vi "Take Measurement.vi"(8 "error in (no error)":errorcluster, 11 "SweepControl in":refnum<class "Sweep Control.lvclass">) -> (0 "error out":errorcluster, 3 "SweepControl":refnum<class "Sweep Control.lvclass">)   [LabVIEW 2019, in "Sweep Control.lvclass"]
uses:
  Sweep Control.lvclass
  Sweep Control.lvclass/Sweep Control.ctl
  <userlib>/LevyLab/Transport/Transport/Transport.lvclass/Transport.ctl
  <userlib>/LevyLab/Transport/Transport/Transport.lvclass
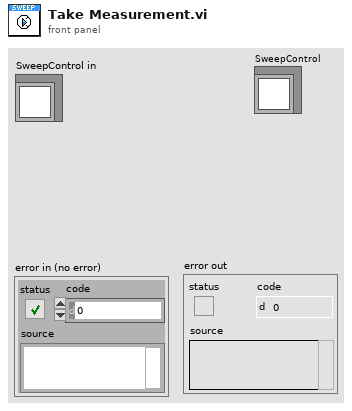
[diagram p1: front panel]
types:
  T1 = typedef "Sweep Control.lvclass/Enum - Experiments.ctl" = enum16{"Lockin_time", "Lockin_sweep", "Lockin_DelayLine"}
  T2 = typedef "Transport.lvclass/Lockin_Sweep JSON--Cluster.ctl" = cluster{"Sweep Time (s)":dbl, "Initial Wait (s)":dbl, "Return to Start":bool, "Sweep Channels":T3, "Sweep Tables":cluster{"Ch":i32, "Table":dbl[]}[]}
  T3 = typedef "Instrument.DAQ.lvclass/Sweep.Channel--Cluster--Array.ctl" = T4[]
  T4 = typedef "Instrument.DAQ.lvclass/Sweep.Channel--Cluster.ctl" = cluster{"Enable?":bool, "Channel":u16, "Start":dbl, "End":dbl, "Pattern":T5, "Table":dbl[]}
  T5 = typedef "Instrument.DAQ.lvclass/Sweep.Pattern--Enum.ctl" = enum16{"Ramp /", "Ramp /\\", "Smooth Ramp _/", "Smooth Ramp _/\\_", "Table"}
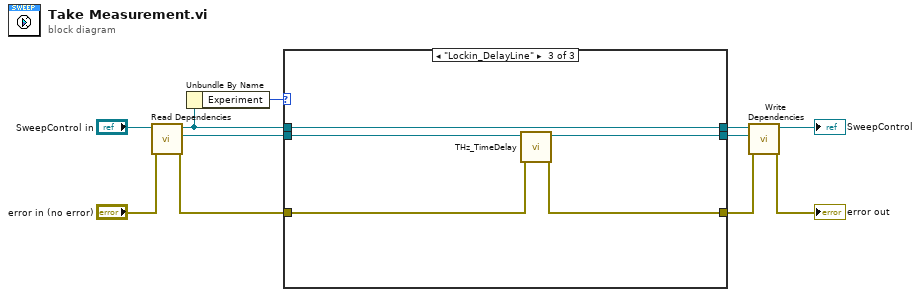
[diagram p0: block diagram]
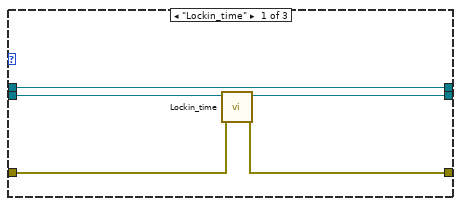
[diagram p2: hidden frame]
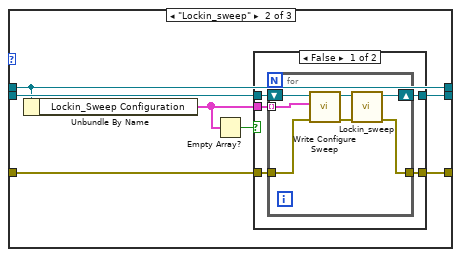
[diagram p3: hidden frame]
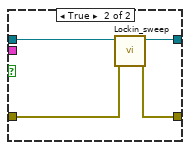
[diagram p4: hidden frame]
diagram:
  n1 = call "Read Dependencies.vi"("error in (no error)"="error in (no error)", "SweepControl in"="SweepControl in") -> ("error out"=w8:errorcluster, "Transport"=w6:refnum<class "Transport.lvclass">, "SweepControl out"=w7:refnum<class "Sweep Control.lvclass">)  [unwired: 7 in]
  n2 = Unbundle By Name(w7) -> ("Experiment"=w11:T1)
  n3 = case shown="\"Lockin_DelayLine\"" w11 {
    tunnel: w8 -> [w13 w18 w41]
    tunnel: w6 -> [w16 w23 w44]
    tunnel: [w12 w22 w40] -> w2
    tunnel: [w15 w21 w43] -> w4
    tunnel: w7 -> [w14 w19 w42]
    tunnel: [w14 w19 w42] -> w5
    frame "Lockin_time" {
      n4 = call <userlib>:"Lockin_time.vi"("error in (no error)"=w13, "Transport"=w16) -> ("error out"=w12:errorcluster, "Transport out"=w15:refnum<class "Transport.lvclass">)  [unwired: 8 in]
    }
    frame "Lockin_sweep" {
      n5 = Unbundle By Name(w19) -> ("Lockin_Sweep Configuration"=w17:T2[])
      n6 = Empty Array?(array=w17) -> (empty?=w20:bool)
      n7 = case shown="False" w20 {
        tunnel: w18 -> [w28 w37]
        tunnel: w23 -> [w27 w39]
        tunnel: [w26 w36] -> w22
        tunnel: [w25 w38] -> w21
        tunnel: w17 -> [w24 _]
        frame False {
          n8 = for {
            tunnel: w28 -> [w30]
            tunnel: [w35] -> w26
            tunnel: w24 -> [w29] mode=indexing
            shift-right: [w34] -> w25
            shift-left: w27 -> [w33]
            n9 = call <userlib>:"Write Configure Sweep.vi"("error in (no error)"=w30, "Lockin_Sweep"=w29, "Transport in"=w33) -> ("error out"=w31:errorcluster, "Transport out"=w32:refnum<class "Transport.lvclass">)  [unwired: 7 in]
            n10 = call <userlib>:"Lockin_sweep.vi"("Transport"=w32, "error in (no error)"=w31) -> ("Transport out"=w34:refnum<class "Transport.lvclass">, "error out"=w35:errorcluster)  [unwired: 7 in]
          }
        }
        frame True {
          n11 = call <userlib>:"Lockin_sweep.vi"("Transport"=w39, "error in (no error)"=w37) -> ("Transport out"=w38:refnum<class "Transport.lvclass">, "error out"=w36:errorcluster)  [unwired: 7 in]
        }
      }
    }
    frame "Lockin_DelayLine" {
      n12 = call <userlib>:"THz_TimeDelay.vi"("error in (no error)"=w41, "Transport"=w44) -> ("error out"=w40:errorcluster, "Transport out"=w43:refnum<class "Transport.lvclass">)  [unwired: 8 in]
    }
  }
  n13 = call "Write Dependencies.vi"("error in (no error)"=w2, "Transport"=w4, "SweepControl in"=w5) -> ("error out"=→"error out":errorcluster, "SweepControl out"=→"SweepControl":refnum<class "Sweep Control.lvclass">)  [unwired: 7 in]
